vi "AI RT FIFO.vi"(0 "Data IN":dbl[](array[numeric]), 1 "Mode":T1=enum."Delete", 7 "Buffer Size":i32=10, 9 "# of elements":i32=1, 11 "Error IN":errorcluster) -> (4 "Data OUT":dbl[][](array[numeric]), 6 "Empty?":bool, 15 "Error OUT":errorcluster)   [LabVIEW 2019]
uses:
  Controls/Stream RT FIFO Mode.ctl
panel:
  out "# elements":u32
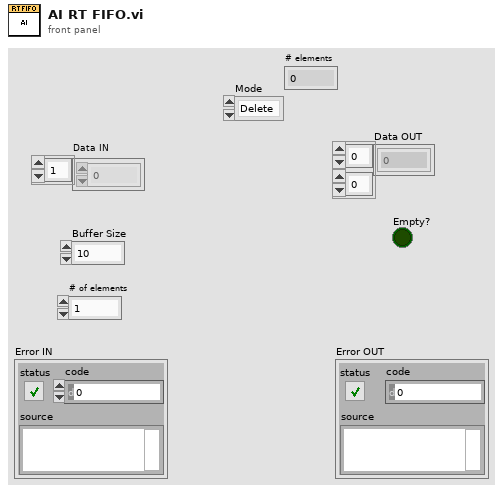
[diagram p1: front panel]
types:
  T1 = typedef "Stream RT FIFO Mode.ctl" = enum16{"Create", "Write", "Read", "Delete"}
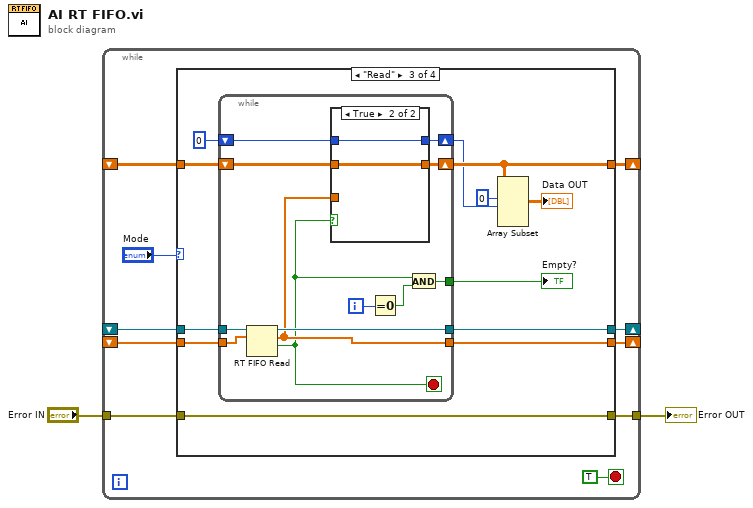
[diagram p0: block diagram]
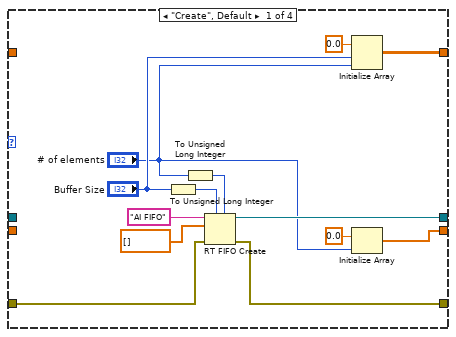
[diagram p2: hidden frame]
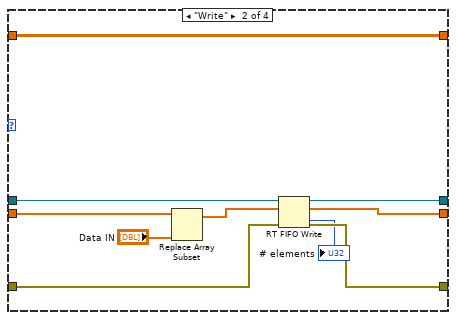
[diagram p3: hidden frame]
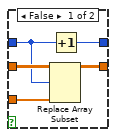
[diagram p4: hidden frame]
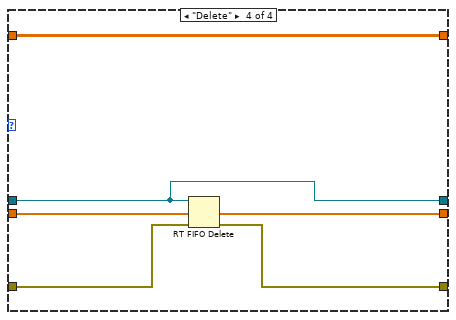
[diagram p5: hidden frame]
diagram:
  n1 = while {
    shift-right: [w10] -> _
    shift-left: _ -> [w9]
    tunnel: "Error IN" -> [w8]
    tunnel: [w7] -> w1
    shift-right: [w6] -> _
    shift-left: _ -> [w5]
    shift-right: [w4] -> _
    shift-left: _ -> [w3]
    stop <- TRUE stop-if-true
    n2 = case shown="\"Read\"" "Mode" {
      tunnel: [w24 w33 w44 w70] -> w10
      tunnel: w9 -> [_ w34 w45 w70]
      tunnel: w8 -> [w20 w29 w46 w68]
      tunnel: [w19 w28 w46 w67] -> w7
      tunnel: [w21 w30 w42 w69] -> w6
      tunnel: w5 -> [_ w32 w43 w69]
      tunnel: [w13 w27 w39 w66] -> w4
      tunnel: w3 -> [_ w27 w40 w66]
      frame "Create", Default {
        n3 = To Unsigned Long Integer(number="Buffer Size") -> (unsigned 32bit integer=w14:u32)
        n4 = To Unsigned Long Integer(number="# of elements") -> (unsigned 32bit integer=w18:u32)
        n5 = RT FIFO Create(0:"AI FIFO" ("name (unnamed)"), 1:dbl[] [], 3:w20, 4:w14, 6:w18) -> (8:w24:refnum<k33>, 11:w19:errorcluster)  [unwired: 3 in, 1 out]
        n6 = Initialize Array(0.0, "Buffer Size", "# of elements") -> (w13:dbl[][])
        n7 = Initialize Array(0.0, "# of elements") -> (w21:dbl[])
      }
      frame "Write" {
        n8 = Replace Array Subset(array=w32, new element="Data IN") -> (w30:dbl[])  [unwired: 1 in]
        n9 = RT FIFO Write(0:w34, 1:w30, 3:w29) -> (7:→"# elements":u32, 8:w33:refnum<k33>, 11:w28:errorcluster)  [unwired: 2 in, 1 out]
      }
      frame "Read" {
        n10 = while {
          tunnel: w45 -> [w58]
          tunnel: [w57] -> w44
          tunnel: w43 -> [w56]
          tunnel: [w51] -> w42
          shift-right: [w54] -> w37
          shift-left: 0 -> [w55]
          shift-right: [w52] -> w39
          shift-left: w40 -> [w53]
          tunnel: [w47] -> w35
          i -> [w49]
          stop <- w50 stop-if-true
          n11 = RT FIFO Read(0:w58, 1:w56) -> (8:w57:refnum<k33>, 9:w51:dbl[], 10:w50:bool)  [unwired: 2 in, 2 out]
          n12 = case shown="True" w50 {
            tunnel: w55 -> [w60 w65]
            tunnel: [w63 w65] -> w54
            tunnel: w53 -> [w62 w64]
            tunnel: [w61 w64] -> w52
            tunnel: w51 -> [w59 _]
            frame False {
              n13 = Replace Array Subset(array=w62, new element=w59, index (row)=w60) -> (w61:dbl[][])  [unwired: 1 in]
              n14 = Increment(x=w60) -> (x+1=w63:i32)
            }
            frame True {
            }
          }
          n15 = Equal To 0?(x=w49) -> (x = 0?=w48:bool)
          n16 = And(x=w50, y=w48) -> (x .and. y?=w47:bool)
        }
        "Empty?" <- w35
        n17 = Array Subset(array=w39, index (row)=0 ("index"), length (row)=w37) -> (→"Data OUT":dbl[][])  [unwired: 2 in]
      }
      frame "Delete" {
        n18 = RT FIFO Delete(0:w70, 3:w68) -> (11:w67:errorcluster)  [unwired: 1 in]
      }
    }
  }
  "Error OUT" <- w1
